vi "Close.vi"(8 "error in (no error)":errorcluster, 11 "Chroma190020 HiPOT in":refnum<class "Chroma190020 HiPOT.lvclass">) -> (0 "error out":errorcluster, 3 "Chroma190020 HiPOT out":refnum<class "Chroma190020 HiPOT.lvclass">)   [LabVIEW 2021, in "Concrete.lvlib" / "Chroma190020 HiPOT.lvclass"]
uses:
  Chroma190020 HiPOT.lvclass
  Chroma190020 HiPOT.lvclass/Chroma190020 HiPOT.ctl
  Harware Abstraction/AnalogIO/AIO.lvclass
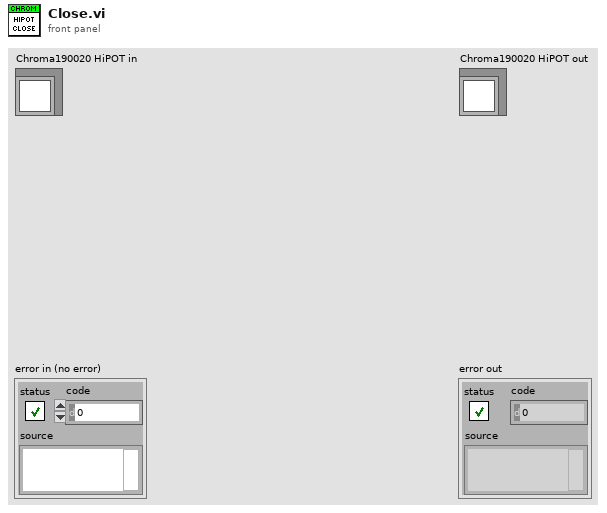
[diagram p1: front panel]
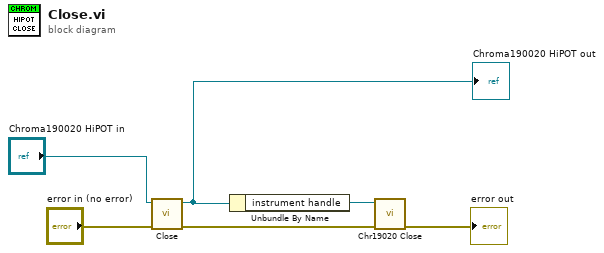
[diagram p0: block diagram]
diagram:
  n1 = call-parent "Close.vi"("error in (no error)"="error in (no error)", "Instrument in"="Chroma190020 HiPOT in") -> ("error out"=w4:errorcluster, "Instrument out"=w2:refnum<class "Chroma190020 HiPOT.lvclass">)  [unwired: 8 in]
  "Chroma190020 HiPOT out" <- w2
  n2 = Unbundle By Name(w2) -> ("instrument handle"=w1:refnum<k15>)
  n3 = call <instrlib>:"Chr19020 Close.vi"("error in (no error)"=w4, "instrument handle"=w1) -> ("error out"=→"error out":errorcluster)  [unwired: 9 in]
